vi "Verify Acquisition.vi"(8 "error in (no error)":errorcluster, 11 "CCDCamera in":refnum<class "Simulated_CCD_Camera.lvclass">) -> (0 "error out":errorcluster, 2 "Acquiring":bool, 3 "CCDCamera out":refnum<class "Simulated_CCD_Camera.lvclass">)   [LabVIEW 2018, in "Simulated_CCD_Camera.lvclass"]
uses:
  Simulated_CCD_Camera.lvclass
  Simulated_CCD_Camera.lvclass/Simulated_CCD_Camera.ctl
  Interface/Interface.lvclass/Interface.ctl
  Interface/Interface.lvclass
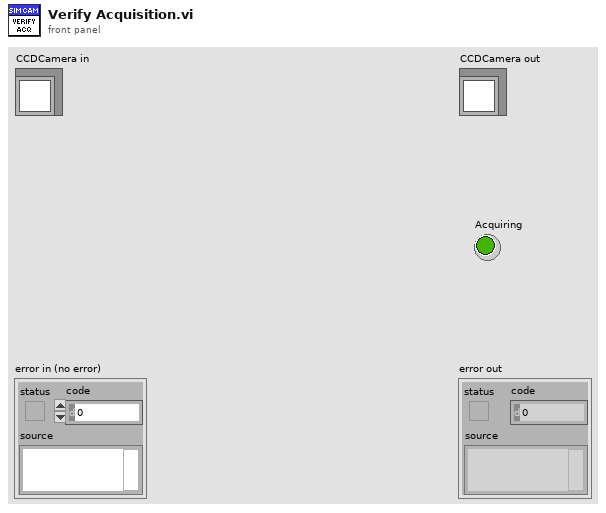
[diagram p1: front panel]
types:
  T1 = typedef "Shutter_mode typedef.ctl" = enum16{"Auto", "Open", "Close", "N/A (3)", "Open FVB Series", "Open Any Series"}
  T2 = typedef "ReadMode_mode typedef.ctl" = enum16{"Full Vertical Binning", "Multi-Track", "Random-Track", "Single-Track", "Image"}
  T3 = typedef "AcquisitionMode_mode typedef.ctl" = enum16{"Reserved (0)", "Single Scan", "Accumulate", "Kinetics", "Fast Kinetics", "Run Till Abort", "Reserved (6)", "Reserved (7)", "Reserved (8)", "Time Delayed Integration"}
  T4 = cluster{"EXPTIME":sgl, "PREAMP":enum16{"Gain 1", "Gain 2"}, "READOUT_RATE":enum16{"30 MHz", "20 MHz", "10 MHz", "1 MHz"}, "EM_GAIN":u16, "VBIN":u16, "INITIAL_LINE":u16, "INITIAL_COLUMN":u16, "FINAL_LINE":u16, "FINAL_COLUMN":u16, "#FRAMES":u32, "#CUBES":u32, "TRIGGER_MODE":enum16{"Internal", "External", "N/A", "N/A_1", "N/A_2", "N/A_3", "External Start"}, "HBIN":u16, "SHUTTER_TTL":enum16{"TTL Low", "TTL High"}, "SHUTTER_MODE":T1, "SHUTTER_OPENING_TIME":u16, "SHUTTER_CLOSING_TIME":u16, "VERTICAL_SHIFT_SPEED":u16, "READ_MODE":T2, "FRAME_TRANSFER":bool, "VERTICAL_CLOCK_VOLTAGE":enum16{"0", "+1", "+2", "+3", "+4"}, "ACQUISITION_MODE":T3, "AD_CHANNEL":u16, "EM_MODE":enum16{"Electron Multiplying", "Conventional"}, "Error In":errorcluster}
  T5 = cluster{"CUBE_EXPOSURE_TIME":sgl, "CUBES_DONE":u16, "LAST_IMAGE_NAME":string, "DISK_SPACE":u16, "FRAMES_DONE":u16, "CCD_STATUS":string, "CURRENT_TEMPERATURE":i16, "TEMPERATURE_STATUS":string, "FRAME_EXPOSURE_TIME":u16, "CCD_ON_OFF":bool, "SERIAL_NUMBER":u16, "ACQUIRING":bool}
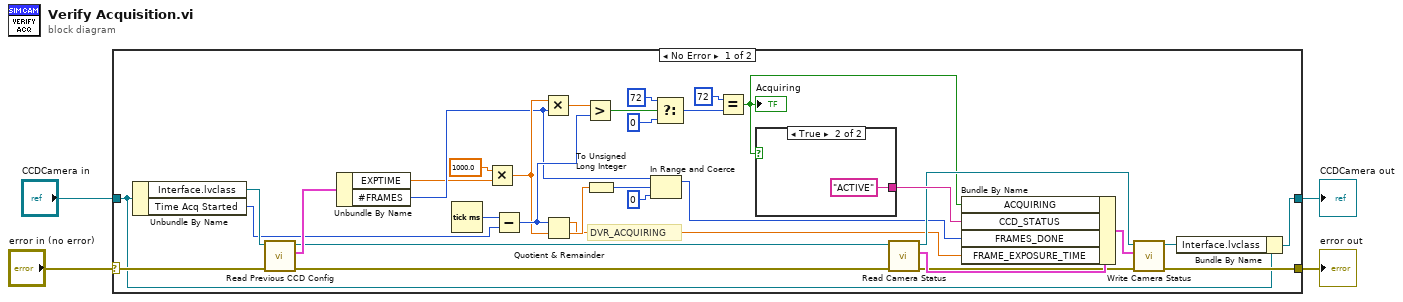
[diagram p0: block diagram]
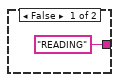
[diagram p2: hidden frame]
diagram:
  n1 = case shown="No Error" "error in (no error)" {
    selector: "error in (no error)" -> [w19 w41]
    tunnel: [w15 w41] -> w1
    tunnel: [w8 w40] -> w2
    tunnel: "CCDCamera in" -> [w10 w40]
    frame No Error {
      # "DVR_ACQUIRING"
      n2 = Unbundle By Name(w10) -> ("Interface.lvclass"=w23:refnum<class "Interface.lvclass">, "Time Acq Started"=w20:u32)
      n3 = call "Read Previous CCD Config.vi"("error in (no error)"=w19, "Interface in"=w23) -> ("error out"=w13:errorcluster, "Previous CCD Config"=w24:T4, "Interface out"=w12:refnum<class "Interface.lvclass">)  [unwired: 7 in]
      n4 = Unbundle By Name(w24) -> ("EXPTIME"=w21:sgl, "#FRAMES"=w22:u32)
      n5 = Tick Count (ms)() -> (millisecond timer value=w36:u32)
      n6 = Multiply(x=1000.0, y=w21) -> (x*y=w25:dbl)
      n7 = Subtract(x=w36, y=w20) -> (x-y=w31:u32)
      n8 = Multiply(x=w25, y=w22) -> (x*y=w26:dbl)
      n9 = Quotient & Remainder(x=w31, y=w25) -> (x-y*floor(x/y)=w5:dbl, floor(x/y)=w32:dbl)
      n10 = Greater?(x=w26, y=w31) -> (0:w35:bool)
      n11 = To Unsigned Long Integer(number=w32) -> (unsigned 32bit integer=w28:u32)
      n12 = In Range and Coerce(upper limit=w22, x=w28, lower limit=u32 0) -> (coerced(x)=w7:u32)  [unwired: 1 out]
      n13 = Select(t=72, s=w35, f=0) -> (s? t:f=w30:i32)
      n14 = Equal?(x=72, y=w30) -> (x = y?=w6:bool)
      "Acquiring" <- w6
      n15 = case shown="True" w6 {
        tunnel: ["READING" "ACTIVE"] -> w16
        frame False {
        }
        frame True {
        }
      }
      n16 = call "Read Camera Status.vi"("error in (no error)"=w13, "Interface in"=w12) -> ("error out"=w14:errorcluster, "Camera Status"=w18:T5, "Interface out"=w11:refnum<class "Interface.lvclass">)  [unwired: 7 in]
      n17 = Bundle By Name(cluster=w18, "ACQUIRING"=w6, "CCD_STATUS"=w16, "FRAMES_DONE"=w7, "FRAME_EXPOSURE_TIME"=w5) -> (w17:T5)
      n18 = call "Write Camera Status.vi"("error in (no error)"=w14, "Camera Status"=w17, "Interface in"=w11) -> ("error out"=w15:errorcluster, "Interface out"=w9:refnum<class "Interface.lvclass">)  [unwired: 7 in]
      n19 = Bundle By Name(cluster=w10, "Interface.lvclass"=w9) -> (w8:refnum<class "Simulated_CCD_Camera.lvclass">)
    }
    frame Error {
    }
  }
  "error out" <- w1
  "CCDCamera out" <- w2
